vi "ADF5355.vi"(8 "Error_In":errorcluster) -> (0 "Error_Out":errorcluster)   [LabVIEW 2018]
uses:
  SP9500/Types/RFU.ctl
  SP9500/Types/RF.ctl
  SP9500/Types/RF_Ver.ctl
  SP9500/Types/LO.ctl
  <vilib>/gmath/NI_Gmath.lvlib
panel:
  out "?":bool
  out "VISA_Rsrc_Out":refnum<visa-resource-name>
  in  "Auto_Sel_Rsrc?":bool=TRUE
  in  "VISA_Rsrc_In":refnum<visa-resource-name>
  in  "LO":T1
  in  "RF_Ver":T2
  in  "RF":T3 items=["RF_0", "RF_1", "RF_2", "RF_3"]
  out "Registers_Rd":u32[](array[numeric]) format="%08x"
  in  "RFU":T4
  in  "Update Freq?":bool=TRUE
  in  "MuxOut":u32(ring)=6 items=["Three-State Output", "DV(DD)", "DGND", "R Divider Output", "N Divider Output", "Analog Lock Detect", "Digital Lock Detect", "Reseved"]
  in  "Current Setting(mA)":u32(ring) items=["0.31", "0.63", "0.94", "1.25", "1.56", "1.88", "2.19", "2.50", "2.81", "3.13", "3.44", "3.75", "4.06", "4.38", "4.69", "5.00"]
  in  "SD Load Reset":u32(ring) items=["On Register0 Update", "Disabled"]
  in  "Reference Doubler":bool
  in  "RDIV2":bool
  in  "Double Buff":bool
  in  "Ref Mode":u32(ring) items=["Single", "Diff"]
  in  "Mux Logic":u32(ring)=1 items=["1.8V", "3.3V"]
  in  "PD Polarity":u32(ring)=1 items=["Negative", "Positive"]
  in  "Counter Reset":bool=TRUE
  in  "CP Three State":bool
  in  "Power Down(PD)":bool
  in  "Phase Resync":bool
  in  "Phase Adjust":bool
  in  "Phase Value(24bit)":u32=1 max=4095
  in  "Prescaler":u32(ring) items=["4/5", "8/9"]
  in  "Autocal":bool=TRUE
  in  "R Counter(1-1023)":u32=1 min=1 max=1023 step=1
  in  "Reference Divider(F)":bool
  in  "Reference Doubler(T)":bool
  in  "Reference Frequency":u32=100000000 format="%3.3p"
  in  "VCO Frequency":u64=10000000 format="%3.9p"
  in  "Resync Clock(0-65535)":u32=20000 max=65535 step=1
  in  "ADC Clock Divider":u32=150 min=1 max=255 step=1
  in  "ADC Conversion":bool=TRUE
  in  "ADC Enable":bool=TRUE
  in  "VCO Band Division(1-255)":u32=40 min=1 max=255 step=1
  in  "Timeout":u32=200 min=1 max=1023 step=1
  in  "Automatic Level Timeout":u32(ring)=30 items=["1", "2", "3", "4", "5", "6", "7", "8", "9", "10", "11", "12", "13", "14", "15", "16", "17", "18", "19", "20", "21", "22", "23", "24", "25", "26", "27", "28", "29", "30", "31"]
  in  "Synthesizer Lock Timeout":u32(ring)=21 items=["1", "2", "3", "4", "5", "6", "7", "8", "9", "10", "11", "12", "13", "14", "15", "16", "17", "18", "19", "20", "21", "22", "23", "24", "25", "26", "27", "28", "29", "30", "31"]
  in  "LeSync":u32(ring)=1 items=["Disable", "Le Synced To Refin"]
  in  "LD Cycle Count":u32(ring) items=["1024", "2048", "4096", "8192"]
  in  "LOL Mode":bool
  in  "Frac-N LD Precision":u32(ring)=3 items=["5.0ns", "6.0ns", "8.0ns", "12.0ns"]
  in  "LD Mode":u32(ring) items=["Fractional-N", "Integer-N(2.9ns)"]
  in  "Gated Bleed":bool
  in  "Negative Bleed":bool=TRUE
  in  "Feedback Select":u32(ring)=1 items=["Divided", "Fundamental"]
  in  "RF Divider Select":u32(ring) items=["÷1", "÷2", "÷4", "÷8", "÷16", "÷32", "÷64"]
  in  "Charge Pump Bleed Current":u32=5 min=1 max=255 step=1
  in  "MTLD":u32(ring) items=["MUTE Disabled", "MUTE Enabled"]
  in  "RF(Out)B":u32(ring)=1 items=["ON", "OFF"]
  in  "RF(Out)A+ / RF(OUT)A-":bool=TRUE
  in  "RF Output Power":u32(ring)=3 items=["-4dBm", "-1dBm", "+2dBm", "+5dBm"]
  out "FRAC2":u32
  out "MOD2":u32
  out "MOD1":u32
  out "FRAC1":u32
  out "INT":u32
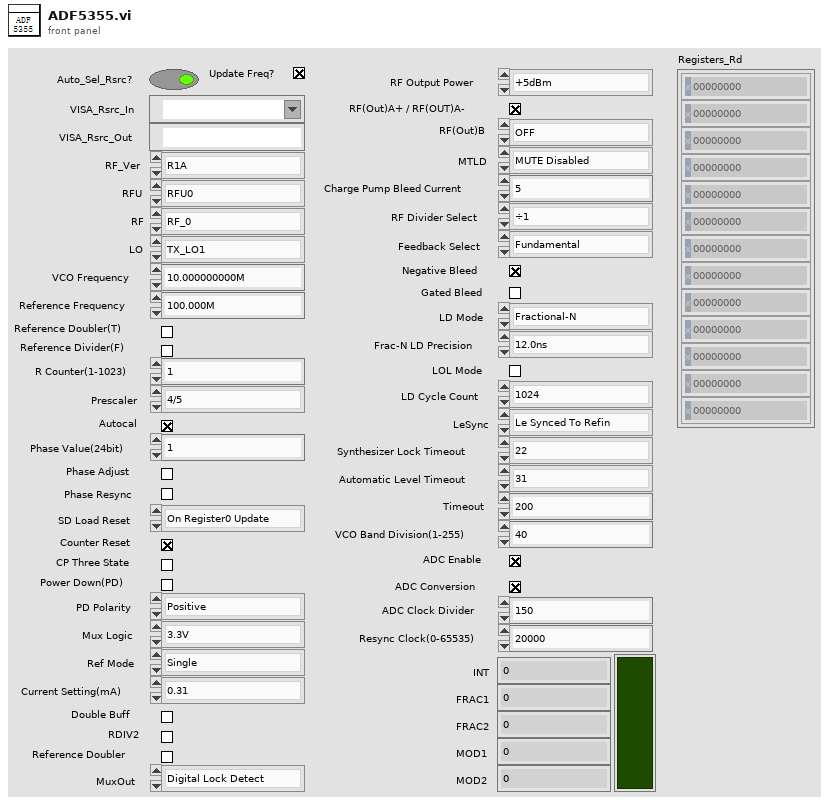
[diagram p1: front panel]
types:
  T1 = typedef "LO.ctl" = enum16{"TX_LO1", "TX_LO2", "TX_LO3", "RX_LO1", "RX_LO2", "RX_LO3"}
  T2 = typedef "RF_Ver.ctl" = enum16{"R1A", "R1B", "R1C", "R1D", "R1E", "R1F"}
  T3 = typedef "RF.ctl" = u16
  T4 = typedef "RFU.ctl" = enum8{"RFU0", "RFU1", "RFU2", "RFU3", "RFU4"}
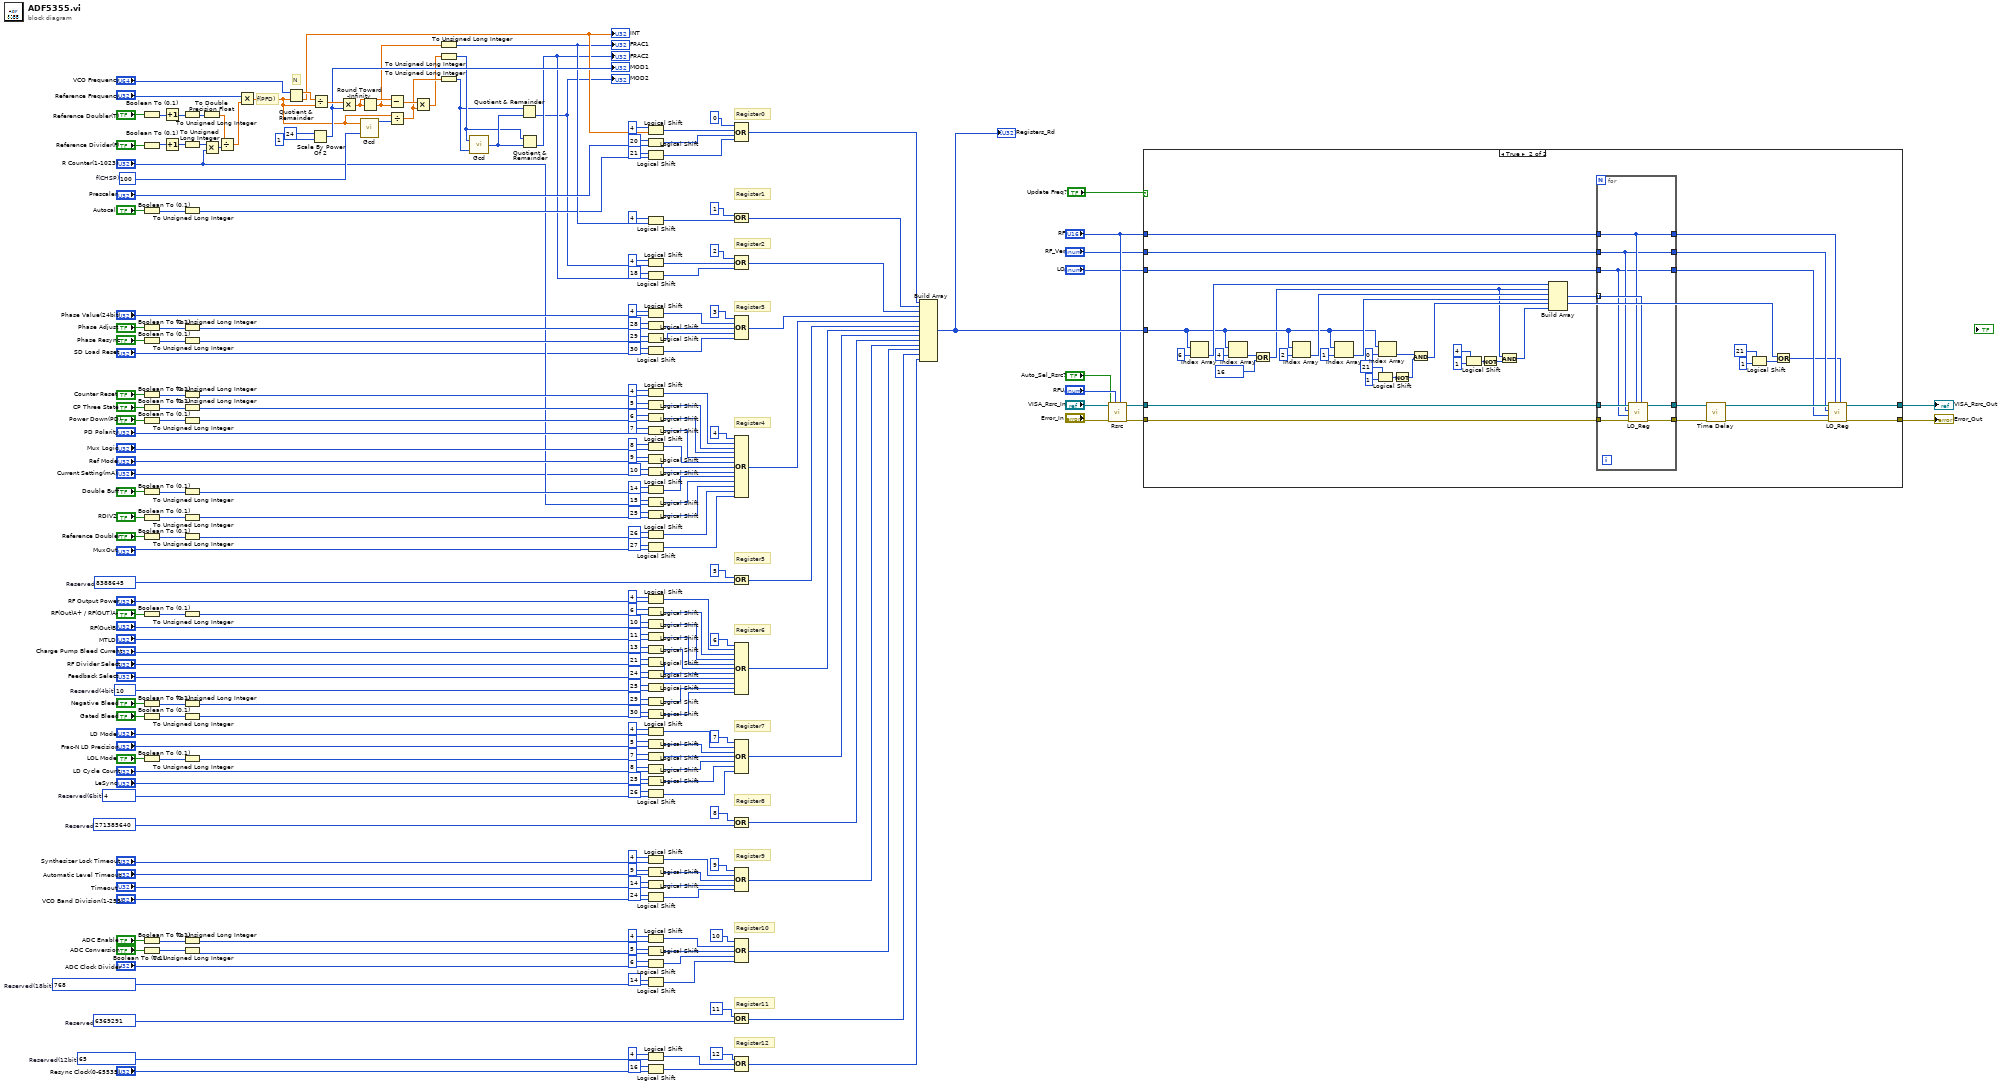
[diagram p0: block diagram]
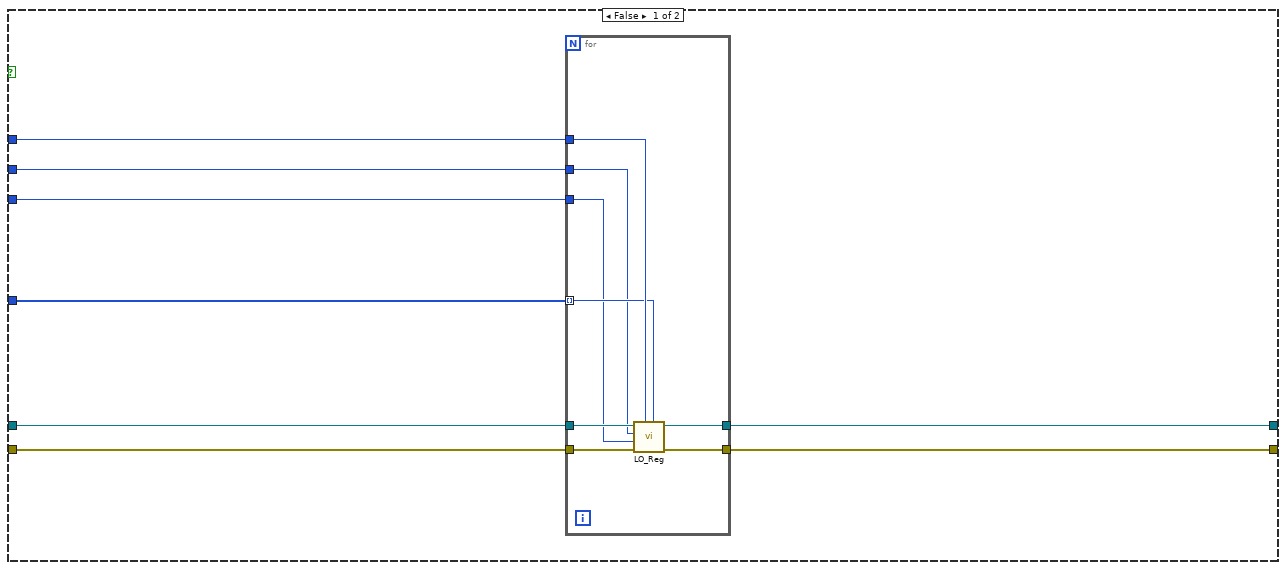
[diagram p2: hidden frame]
diagram:
  w38 = u32 10  # Reserved(4bit)
  w40 = u32 4  # Reserved(6bit)
  w43 = u32 768  # Reserved(18bit)
  w46 = u32 65  # Reserved(12bit)
  w55 = u32 6369291  # Reserved
  w85 = u32 271385640  # Reserved
  w137 = u32 8388645  # Reserved
  w230 = 100  # f(CHSP)
  # "Register12"
  # "Register11"
  # "Register10"
  # "Register9"
  # "Register8"
  # "Register7"
  # "Register6"
  # "Register5"
  # "Register4"
  # "Register3"
  # "Register2"
  # "Register1"
  # "Register0"
  # "N"
  # "f(PFD)"
  n1 = Boolean To (0,1)(Boolean="Reference Doubler(T)") -> (0, 1=w244:i16)
  n2 = Boolean To (0,1)(Boolean="Reference Divider(F)") -> (0, 1=w240:i16)
  n3 = Boolean To (0,1)(Boolean="Autocal") -> (0, 1=w201:i16)
  n4 = Boolean To (0,1)(Boolean="Phase Adjust") -> (0, 1=w202:i16)
  n5 = Boolean To (0,1)(Boolean="Phase Resync") -> (0, 1=w199:i16)
  n6 = Boolean To (0,1)(Boolean="Counter Reset") -> (0, 1=w170:i16)
  n7 = Boolean To (0,1)(Boolean="CP Three State") -> (0, 1=w172:i16)
  n8 = Boolean To (0,1)(Boolean="Power Down(PD)") -> (0, 1=w173:i16)
  n9 = Boolean To (0,1)(Boolean="Double Buff") -> (0, 1=w165:i16)
  n10 = Boolean To (0,1)(Boolean="RDIV2") -> (0, 1=w164:i16)
  n11 = Boolean To (0,1)(Boolean="Reference Doubler") -> (0, 1=w161:i16)
  n12 = Boolean To (0,1)(Boolean="RF(Out)A+ / RF(OUT)A-") -> (0, 1=w136:i16)
  n13 = Boolean To (0,1)(Boolean="Negative Bleed") -> (0, 1=w133:i16)
  n14 = Boolean To (0,1)(Boolean="Gated Bleed") -> (0, 1=w132:i16)
  n15 = Boolean To (0,1)(Boolean="LOL Mode") -> (0, 1=w102:i16)
  n16 = Boolean To (0,1)(Boolean="ADC Enable") -> (0, 1=w70:i16)
  n17 = Boolean To (0,1)(Boolean="ADC Conversion") -> (0, 1=w67:i16)
  n18 = Increment(x=w244) -> (x+1=w242:i16)
  n19 = Increment(x=w240) -> (x+1=w241:i16)
  n20 = To Unsigned Long Integer(number=w242) -> (unsigned 32bit integer=w22:u32)
  n21 = To Unsigned Long Integer(number=w241) -> (unsigned 32bit integer=w238:u32)
  n22 = To Unsigned Long Integer(number=w201) -> (unsigned 32bit integer=w200:u32)
  n23 = To Unsigned Long Integer(number=w202) -> (unsigned 32bit integer=w189:u32)
  n24 = To Unsigned Long Integer(number=w199) -> (unsigned 32bit integer=w188:u32)
  n25 = To Unsigned Long Integer(number=w170) -> (unsigned 32bit integer=w168:u32)
  n26 = To Unsigned Long Integer(number=w172) -> (unsigned 32bit integer=w182:u32)
  n27 = To Unsigned Long Integer(number=w173) -> (unsigned 32bit integer=w183:u32)
  n28 = To Unsigned Long Integer(number=w165) -> (unsigned 32bit integer=w150:u32)
  n29 = To Unsigned Long Integer(number=w164) -> (unsigned 32bit integer=w148:u32)
  n30 = To Unsigned Long Integer(number=w161) -> (unsigned 32bit integer=w147:u32)
  n31 = To Unsigned Long Integer(number=w136) -> (unsigned 32bit integer=w111:u32)
  n32 = To Unsigned Long Integer(number=w133) -> (unsigned 32bit integer=w105:u32)
  n33 = To Unsigned Long Integer(number=w132) -> (unsigned 32bit integer=w104:u32)
  n34 = To Unsigned Long Integer(number=w102) -> (unsigned 32bit integer=w88:u32)
  n35 = To Unsigned Long Integer(number=w70) -> (unsigned 32bit integer=w59:u32)
  n36 = To Unsigned Long Integer(number=w67) -> (unsigned 32bit integer=w58:u32)
  n37 = To Double Precision Float(number=w22) -> (double precision float=w21:dbl)
  n38 = Multiply(x=w238, y="R Counter(1-1023)") -> (x*y=w20:u32)
  n39 = Divide(x=w21, y=w20) -> (x/y=w237:dbl)
  n40 = Multiply(x="Reference Frequency", y=w237) -> (x*y=w229:dbl)
  n41 = Quotient & Remainder(x="VCO Frequency", y=w229) -> (x-y*floor(x/y)=w235:dbl, floor(x/y)=w221:dbl)
  "INT" <- w221
  n42 = Scale By Power Of 2(n=24, x=1) -> (x*2^n=w231:i32)
  "MOD1" <- w231
  n43 = Divide(x=w235, y=w229) -> (x/y=w234:dbl)
  n44 = Multiply(x=w234, y=w231) -> (x*y=w227:dbl)
  n45 = call <vilib>:"Gcd.vi"("y"=w230, "x"=w229) -> ("gcd(x,y)"=w228:i32)
  n46 = Round Toward -Infinity(1:w227) -> (0:w212:dbl)
  n47 = Subtract(x=w227, y=w212) -> (x-y=w226:dbl)
  n48 = Divide(x=w229, y=w228) -> (x/y=w205:dbl)
  n49 = Multiply(x=w226, y=w205) -> (x*y=w204:dbl)
  n50 = To Unsigned Long Integer(number=w212) -> (unsigned 32bit integer=w211:u32)
  "FRAC1" <- w211
  n51 = To Unsigned Long Integer(number=w204) -> (unsigned 32bit integer=w18:u32)
  n52 = To Unsigned Long Integer(number=w205) -> (unsigned 32bit integer=w16:u32)
  n53 = call <vilib>:"Gcd.vi"("y"=w16, "x"=w18) -> ("gcd(x,y)"=w19:i32)
  n54 = Quotient & Remainder(x=w16, y=w19) -> (floor(x/y)=w15:u32)  [unwired: 1 out]
  "MOD2" <- w15
  n55 = Quotient & Remainder(x=w18, y=w19) -> (floor(x/y)=w17:u32)  [unwired: 1 out]
  "FRAC2" <- w17
  n56 = Logical Shift(y=i8 4, x=w221) -> (x << y=w223:u32)
  n57 = Logical Shift(y=i8 20, x="Prescaler") -> (x << y=w224:u32)
  n58 = Logical Shift(y=i8 21, x=w200) -> (x << y=w216:u32)
  n59 = Logical Shift(y=i8 4, x=w211) -> (x << y=w213:u32)
  n60 = Logical Shift(y=i8 4, x=w15) -> (x << y=w208:u32)
  n61 = Logical Shift(y=i8 18, x=w17) -> (x << y=w207:u32)
  n62 = Logical Shift(y=i8 4, x="Phase Value(24bit)") -> (x << y=w193:u32)
  n63 = Logical Shift(y=i8 28, x=w189) -> (x << y=w192:u32)
  n64 = Logical Shift(y=i8 29, x=w188) -> (x << y=w197:u32)
  n65 = Logical Shift(y=i8 30, x="SD Load Reset") -> (x << y=w186:u32)
  n66 = Logical Shift(y=i8 4, x=w168) -> (x << y=w179:u32)
  n67 = Logical Shift(y=i8 5, x=w182) -> (x << y=w180:u32)
  n68 = Logical Shift(y=i8 6, x=w183) -> (x << y=w175:u32)
  n69 = Logical Shift(y=i8 7, x="PD Polarity") -> (x << y=w185:u32)
  n70 = Logical Shift(y=i8 8, x="Mux Logic") -> (x << y=w146:u32)
  n71 = Logical Shift(y=i8 9, x="Ref Mode") -> (x << y=w145:u32)
  n72 = Logical Shift(y=i8 10, x="Current Setting(mA)") -> (x << y=w144:u32)
  n73 = Logical Shift(y=i8 14, x=w150) -> (x << y=w143:u32)
  n74 = Logical Shift(y=i8 15, x="R Counter(1-1023)") -> (x << y=w142:u32)
  n75 = Logical Shift(y=i8 25, x=w148) -> (x << y=w141:u32)
  n76 = Logical Shift(y=i8 26, x=w147) -> (x << y=w140:u32)
  n77 = Logical Shift(y=i8 27, x="MuxOut") -> (x << y=w139:u32)
  n78 = Logical Shift(y=i8 4, x="RF Output Power") -> (x << y=w117:u32)
  n79 = Logical Shift(y=i8 6, x=w111) -> (x << y=w116:u32)
  n80 = Logical Shift(y=i8 10, x="RF(Out)B") -> (x << y=w121:u32)
  n81 = Logical Shift(y=i8 11, x="MTLD") -> (x << y=w113:u32)
  n82 = Logical Shift(y=i8 13, x="Charge Pump Bleed Current") -> (x << y=w127:u32)
  n83 = Logical Shift(y=i8 21, x="RF Divider Select") -> (x << y=w128:u32)
  n84 = Logical Shift(y=i8 24, x="Feedback Select") -> (x << y=w129:u32)
  n85 = Logical Shift(y=i8 25, x=w38) -> (x << y=w36:u32)
  n86 = Logical Shift(y=i8 29, x=w105) -> (x << y=w37:u32)
  n87 = Logical Shift(y=i8 30, x=w104) -> (x << y=w130:u32)
  n88 = Logical Shift(y=i8 4, x="LD Mode") -> (x << y=w97:u32)
  n89 = Logical Shift(y=i8 5, x="Frac-N LD Precision") -> (x << y=w98:u32)
  n90 = Logical Shift(y=i8 7, x=w88) -> (x << y=w93:u32)
  n91 = Logical Shift(y=i8 8, x="LD Cycle Count") -> (x << y=w101:u32)
  n92 = Logical Shift(y=i8 25, x="LeSync") -> (x << y=w91:u32)
  n93 = Logical Shift(y=i8 26, x=w40) -> (x << y=w14:u32)
  n94 = Logical Shift(y=i8 4, x="Synthesizer Lock Timeout") -> (x << y=w79:u32)
  n95 = Logical Shift(y=i8 9, x="Automatic Level Timeout") -> (x << y=w78:u32)
  n96 = Logical Shift(y=i8 14, x="Timeout") -> (x << y=w83:u32)
  n97 = Logical Shift(y=i8 24, x="VCO Band Division(1-255)") -> (x << y=w75:u32)
  n98 = Logical Shift(y=i8 4, x=w59) -> (x << y=w64:u32)
  n99 = Logical Shift(y=i8 5, x=w58) -> (x << y=w65:u32)
  n100 = Logical Shift(y=i8 6, x="ADC Clock Divider") -> (x << y=w60:u32)
  n101 = Logical Shift(y=i8 14, x=w43) -> (x << y=w42:u32)
  n102 = Logical Shift(y=i8 4, x=w46) -> (x << y=w45:u32)
  n103 = Logical Shift(y=i8 16, x="Resync Clock(0-65535)") -> (x << y=w47:u32)
  n104 = Compound Arithmetic op=OR(u32 0 ("value"), w223, w224, w216) -> (w35:u32)
  n105 = Compound Arithmetic op=OR(u32 1 ("value"), w213) -> (w34:u32)
  n106 = Compound Arithmetic op=OR(u32 2 ("value"), w208, w207) -> (w33:u32)
  n107 = Compound Arithmetic op=OR(u32 3 ("value"), w193, w192, w197, w186) -> (w32:u32)
  n108 = Compound Arithmetic op=OR(u32 4 ("value"), w179, w180, w175, w185, w146, w145, w144, w143, w142, w141, w140, w139) -> (w31:u32)
  n109 = Compound Arithmetic op=OR(u32 5 ("value"), w137) -> (w30:u32)
  n110 = Compound Arithmetic op=OR(u32 6 ("value"), w117, w116, w121, w113, w127, w128, w129, w36, w37, w130) -> (w29:u32)
  n111 = Compound Arithmetic op=OR(u32 7 ("value"), w97, w98, w93, w101, w91, w14) -> (w28:u32)
  n112 = Compound Arithmetic op=OR(u32 8 ("value"), w85) -> (w27:u32)
  n113 = Compound Arithmetic op=OR(u32 9 ("value"), w79, w78, w83, w75) -> (w26:u32)
  n114 = Compound Arithmetic op=OR(u32 10 ("value"), w64, w65, w60, w42) -> (w25:u32)
  n115 = Compound Arithmetic op=OR(u32 11 ("value"), w55) -> (w24:u32)
  n116 = Compound Arithmetic op=OR(u32 12 ("value"), w45, w47) -> (w23:u32)
  n117 = Build Array(w35, w34, w33, w32, w31, w30, w29, w28, w27, w26, w25, w24, w23) -> (w7:u32[])
  "Registers_Rd" <- w7
  n118 = call "Rsrc.vi"("RF"="RF", "RFU"="RFU", "Error_In"="Error_In", "Auto_Sel_Rsrc?"="Auto_Sel_Rsrc?", "VISA_Rsrc_In"="VISA_Rsrc_In") -> ("Error_Out"=w10:errorcluster, "VISA_Rsrc_Out"=w11:refnum<visa-resource-name>)  [unwired: 5 in]
  n119 = case shown="True" "Update Freq?" {
    tunnel: w11 -> [w253 w302]
    tunnel: w10 -> [w252 w301]
    tunnel: [w251 w264] -> w1
    tunnel: [w250 w265] -> w2
    tunnel: w7 -> [w249 w275]
    tunnel: "RF" -> [w248 w280]
    tunnel: "RF_Ver" -> [w247 w279]
    tunnel: "LO" -> [w246 w278]
    frame False {
      n120 = for {
        tunnel: w253 -> [w261]
        tunnel: w252 -> [w260]
        tunnel: w249 -> [w258] mode=indexing
        tunnel: [w256] -> w251
        tunnel: [w257] -> w250
        tunnel: w248 -> [w259]
        tunnel: w247 -> [w255]
        tunnel: w246 -> [w254]
        n121 = call "LO_Reg.vi"("Reg_Data"=w258, "RF"=w259, "Error_In"=w260, "LO"=w254, "RF_Ver"=w255, "VISA_Rsrc_In"=w261) -> ("Error_Out"=w256:errorcluster, "VISA_Rsrc_Out"=w257:refnum<visa-resource-name>)  [unwired: 4 in]
      }
    }
    frame True {
      n122 = Index Array(array=w275, index=6) -> (element=w284:u32)
      n123 = Index Array(array=w275, index=4) -> (element=w298:u32)
      n124 = Or(x=w298, y=u32 16) -> (x .or. y?=w262:u32)
      n125 = Index Array(array=w275, index=2) -> (element=w283:u32)
      n126 = Index Array(array=w275, index=1) -> (element=w282:u32)
      n127 = Logical Shift(y=i16 21, x=u32 1) -> (x << y=w291:u32)
      n128 = Index Array(array=w275, index=0) -> (element=w290:u32)
      n129 = Not(x=w291) -> (.not. x?=w289:u32)
      n130 = And(x=w290, y=w289) -> (x .and. y?=w263:u32)
      n131 = Logical Shift(y=i16 4, x=u32 1) -> (x << y=w287:u32)
      n132 = Not(x=w287) -> (.not. x?=w288:u32)
      n133 = And(x=w262, y=w288) -> (x .and. y?=w281:u32)
      n134 = Build Array(w284, w262, w283, w282, w263, w281) -> (w277:u32[])
      n135 = for {
        tunnel: w302 -> [w310]
        tunnel: w301 -> [w309]
        tunnel: w280 -> [w305]
        tunnel: w279 -> [w304]
        tunnel: w278 -> [w303]
        tunnel: w277 -> [w308] mode=indexing
        tunnel: [w307] -> w270
        tunnel: [w306] -> w276
        tunnel: [w305] -> w269
        tunnel: [w304] -> w268
        tunnel: [w303] -> w267
        n136 = call "LO_Reg.vi"("Reg_Data"=w308, "RF"=w305, "Error_In"=w309, "LO"=w303, "RF_Ver"=w304, "VISA_Rsrc_In"=w310) -> ("Error_Out"=w306:errorcluster, "VISA_Rsrc_Out"=w307:refnum<visa-resource-name>)  [unwired: 4 in]
      }
      n137 = call "Time Delay"("error in (no error)"=w276) -> ("error out"=w271:errorcluster)  [unwired: 10 in]
      n138 = Logical Shift(y=i16 21, x=u32 1) -> (x << y=w272:u32)
      n139 = Or(x=w263, y=w272) -> (x .or. y?=w266:u32)
      n140 = call "LO_Reg.vi"("Reg_Data"=w266, "RF"=w269, "Error_In"=w271, "LO"=w267, "RF_Ver"=w268, "VISA_Rsrc_In"=w270) -> ("Error_Out"=w264:errorcluster, "VISA_Rsrc_Out"=w265:refnum<visa-resource-name>)  [unwired: 4 in]
    }
  }
  "Error_Out" <- w1
  "VISA_Rsrc_Out" <- w2
